vi "Eng Mode Password.vi"() -> (6 "Password Match":bool=TRUE)   [LabVIEW 2017]
uses:
  <vilib>/ErrorRing/Error Ring.xnode
panel:
  in  "Panel Close?":bool
  in  "Enter Button":bool
  in  "Password Input":string
  # "Enter Engineering Password"
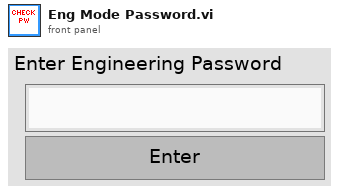
[diagram p1: front panel]
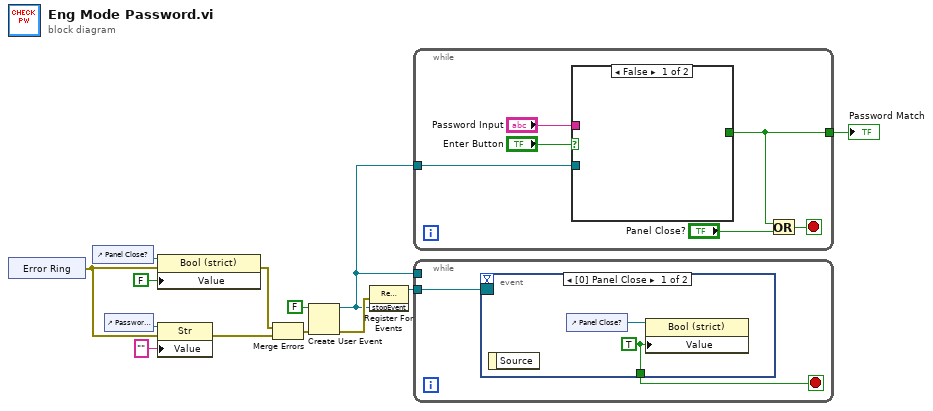
[diagram p0: block diagram]
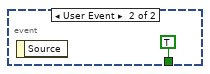
[diagram p2: hidden frame]
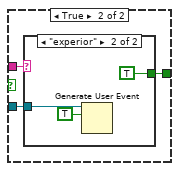
[diagram p3: hidden frame]
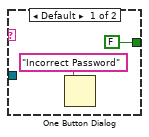
[diagram p4: hidden frame]
diagram:
  n1 = xnode "Error Ring"() -> ("error out"=w6:errorcluster)
  n2 = control-ref of="Panel Close?"() -> (w9:refnum<vi>)
  n3 = control-ref of="Password Input"() -> (w8:refnum<vi>)
  n4 = property class="Bool (strict)"(reference=w9, error in=w6, "Value"=FALSE) -> (error out=w5:errorcluster)  [unwired: 1 out]
  n5 = property class="Str"(reference=w8, error in=w6, "Value"="") -> (error out=w4:errorcluster)  [unwired: 1 out]
  n6 = Merge Errors(w5, w4) -> (w3:errorcluster)
  n7 = Create User Event(user event datatype=FALSE ("stopEvent"), error in=w3) -> (user event=w1:refnum<user-event>, error out=w2:errorcluster)
  n8 = register-events(error in=w2, w1) -> (reference out=w11:refnum<event-registration>)  [unwired: 1 in, 1 out]
  n9 = while {
    tunnel: [w17] -> w13
    tunnel: w1 -> [w14]
    stop <- w16 stop-if-true
    n10 = case shown="False" "Enter Button" {
      tunnel: [_ w22] -> w17
      tunnel: "Password Input" -> [_ w21]
      tunnel: w14 -> [_ w20]
      frame False {
      }
      frame True {
        n11 = case shown="\"experior\"" w21 {
          tunnel: [FALSE TRUE] -> w22
          tunnel: w20 -> [_ w26]
          frame Default {
            n12 = One Button Dialog(message="Incorrect Password") -> ()  [unwired: 1 in, 1 out]
          }
          frame "experior" {
            n13 = Generate User Event(user event=w26, event data cluster=TRUE ("event data")) -> ()  [unwired: 2 in, 2 out]
          }
        }
      }
    }
    n14 = Or(x=w17, y="Panel Close?") -> (x .or. y?=w16:bool)
  }
  "Password Match" <- w13
  n15 = while {
    tunnel: w11 -> [w28]
    tunnel: w1 -> [_]
    stop <- w29 stop-if-true
    n16 = event shown="[0] Panel Close" {
      selector: w28 -> [_ _]
      dyn-events: _ -> [_ _]
      timeout: _ -> [_ _]
      tunnel: [w30 TRUE ("Value")] -> w29
      event Panel Close {
        w30 = TRUE ("Value")
        n17 = event-data() -> ()  [unwired: 1 in, 1 out]
        n18 = control-ref of="Panel Close?"() -> (w31:refnum<vi>)
        n19 = property class="Bool (strict)"(reference=w31, "Value"=w30) -> ()  [unwired: 1 in, 2 out]
      }
      event User Event {
        n20 = event-data() -> ()  [unwired: 1 in, 1 out]
      }
    }
  }
